vi "Run.vi"(7 "Team Index":i32, 8 "Column":i32, 9 "Row":i32, 10 "View":i32[](array[numeric]) caption="View (Team Index, -1: empty)", 11 "Runner in":refnum<class "Rain.lvclass">) -> (0 "Replicated":refnum<class "Square.lvclass">, 1 "Direction":T1, 2 "Action":T2, 3 "Square Out":refnum<class "Square.lvclass">)   [LabVIEW 2020, in "Rain.lvclass"]
uses:
  Rain.lvclass
  C:/dev/IlluminatedG/sol-squarebattle/Square/Square.lvclass
  Square/Square.lvclass
  Type Defs/Action Enum.ctl
  Type Defs/Direction Enum.ctl
  Common/Attack Options.ctl
  SubVIs/Read-Only Globals.vi
  SubVIs/Globals (private).vi
  Common/Find Enemy.vi
  Common/Reverse Direction.vi
  Common/Common.lvlib
  Type Defs/SB Type Defs.lvlib
panel:
  # "NW\nN\nNE\nE\nSE\nS\nSW\nW"
  # "NOTICE - YOU MUST NOT REMOVE THIS NOTICE. PER THE FOLLOWING LICENSE, YOU MAY REPRODUCE THIS SOFTWARE PROVIDED YOU FOLLOW THE TERMS\nOF THE LICENSE.\n\n---BEGIN BSD LICENSE (http://opensource.org/licenses/BSD-2-Clause)---\nCopyright (c) 2015, Endigit, Inc. <robert@endigit.com>\nAll rights reserved.\n\nRedistribution and use in source and binary forms, with or without modification, are permitted provided that the following conditions are met:\n\n1. Redistributions of source code must retain the above copyright notice, this list of conditions and the following disclaimer.\n\n2. Redistributions in binary form must reproduce the above copyright notice, this list of conditions and the following disclaimer in the documentation and/or other \nmaterials provided with the distribution.\n\nTHIS SOFTWARE IS PROVIDED BY THE COPYRIGHT HOLDERS AND CONTRIBUTORS \"AS IS\" AND ANY EXPRESS OR IMPLIED WARRANTIES, INCLUDING, BUT NOT \nLIMITED TO, THE IMPLIED WARRANTIES OF MERCHANTABILITY AND FITNESS FOR A PARTICULAR PURPOSE ARE DISCLAIMED. IN NO EVENT SHALL THE COPYRIGHT \nHOLDER OR CONTRIBUTORS BE LIABLE FOR ANY DIRECT, INDIRECT, INCIDENTAL, SPECIAL, EXEMPLARY, OR CONSEQUENTIAL DAMAGES (INCLUDING, BUT NOT \nLIMITED TO, PROCUREMENT OF SUBSTITUTE GOODS OR SERVICES; LOSS OF USE, DATA, OR PROFITS; OR BUSINESS INTERRUPTION) HOWEVER CAUSED AND ON \nANY THEORY OF LIABILITY, WHETHER IN CONTRACT, STRICT LIABILITY, OR TORT (INCLUDING NEGLIGENCE OR OTHERWISE) ARISING IN ANY WAY OUT OF THE USE \nOF THIS SOFTWARE, EVEN IF ADVISED OF THE POSSIBILITY OF SUCH DAMAGE.\n---END BSD LICENSE---"
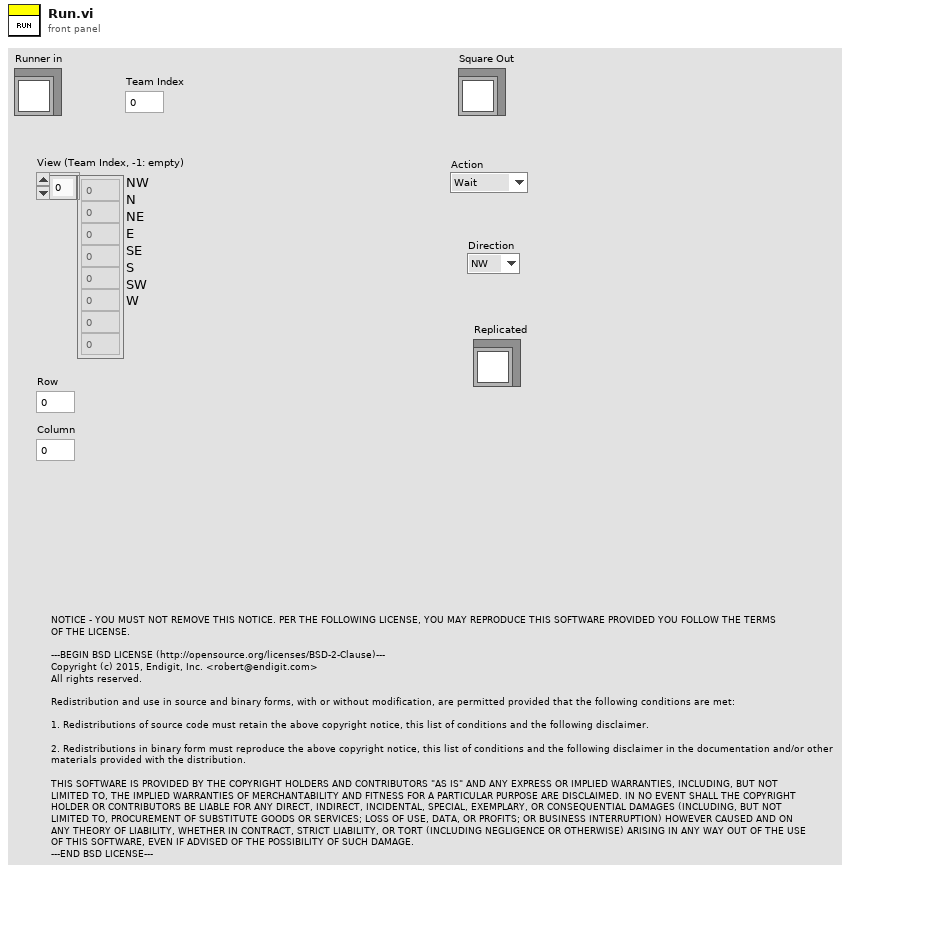
[diagram p1: front panel]
types:
  T1 = typedef "SB Type Defs.lvlib/Direction Enum.ctl" = enum16{"NW", "N", "NE", "E", "SE", "S", "SW", "W"}
  T2 = typedef "SB Type Defs.lvlib/Action Enum.ctl" = enum16{"Wait", "Move", "Attack", "Replicate"}
  T3 = typedef "Common.lvlib/Attack Options.ctl" = enum16{"Attack", "Run", "Distract"}
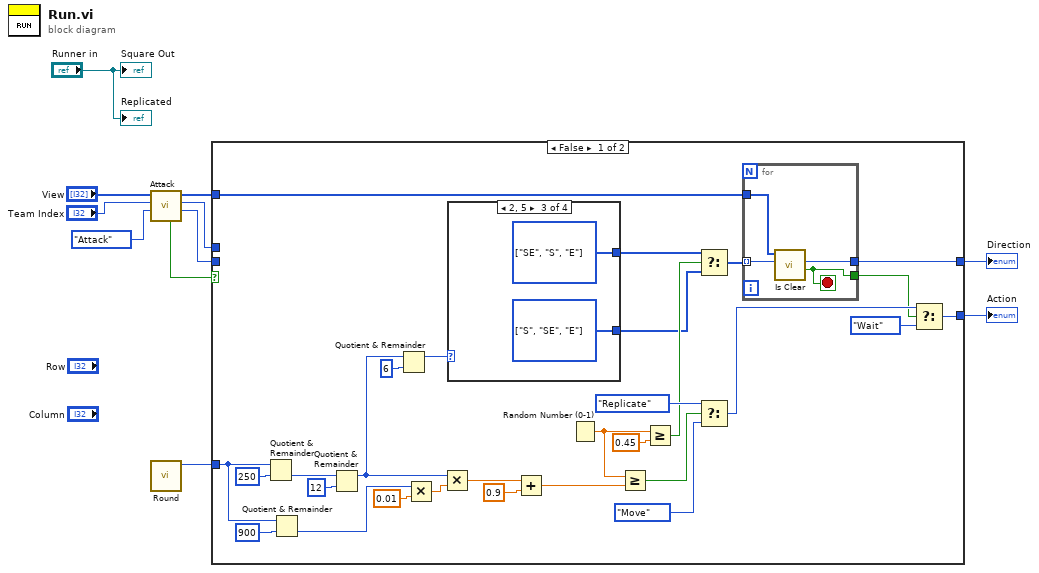
[diagram p0: block diagram]
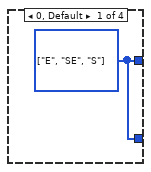
[diagram p2: hidden frame]
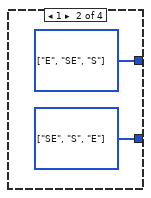
[diagram p3: hidden frame]
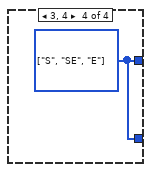
[diagram p4: hidden frame]
diagram:
  n1 = call "Attack.vi"("Attack?"=Attack_Options."Attack" ("Attack"), "Team Index"="Team Index", "View"="View") -> ("Direction"=w10:i32, "Action"=w8:T2, "View"=w6:i32[], "Enemy Found?"=w11:bool)  [unwired: 3 in, 2 out]
  n2 = call "Round.vi"() -> ("Round"=w3:i32)  [unwired: 11 in]
  n3 = case shown="False" w11 {
    tunnel: w10 -> [_ w52]
    tunnel: [w33 w52] -> w9
    tunnel: w8 -> [_ w51]
    tunnel: [w37 w51] -> w7
    tunnel: w6 -> [w34 _]
    tunnel: w3 -> [w16 _]
    frame False {
      n4 = Quotient & Remainder(x=w16, y=250) -> (floor(x/y)=w24:i32)  [unwired: 1 out]
      n5 = Quotient & Remainder(x=w16, y=900) -> (floor(x/y)=w14:i32)  [unwired: 1 out]
      n6 = Quotient & Remainder(x=w24, y=12) -> (x-y*floor(x/y)=w18:i32)  [unwired: 1 out]
      n7 = Quotient & Remainder(x=w18, y=6) -> (x-y*floor(x/y)=w17:i32)  [unwired: 1 out]
      n8 = Multiply(x=w14, y=0.01) -> (x*y=w12:dbl)
      n9 = Multiply(x=w18, y=w12) -> (x*y=w23:dbl)
      n10 = case shown="2, 5" w17 {
        tunnel: [w41 w43 w45 w46] -> w28
        tunnel: [w41 w42 w44 w46] -> w29
        frame 0, Default {
          w41 = T1[] [enum."E", enum."SE", enum."S"] items=["NW", "N", "NE", "E", "SE", "S", "SW", "W"]
        }
        frame 1 {
          w42 = T1[] [enum."SE", enum."S", enum."E"] items=["NW", "N", "NE", "E", "SE", "S", "SW", "W"]
          w43 = T1[] [enum."E", enum."SE", enum."S"] items=["NW", "N", "NE", "E", "SE", "S", "SW", "W"]
        }
        frame 2, 5 {
          w44 = T1[] [enum."S", enum."SE", enum."E"] items=["NW", "N", "NE", "E", "SE", "S", "SW", "W"]
          w45 = T1[] [enum."SE", enum."S", enum."E"] items=["NW", "N", "NE", "E", "SE", "S", "SW", "W"]
        }
        frame 3, 4 {
          w46 = T1[] [enum."S", enum."SE", enum."E"] items=["NW", "N", "NE", "E", "SE", "S", "SW", "W"]
        }
      }
      n11 = Add(x=w23, y=0.9) -> (x+y=w21:dbl)
      n12 = Random Number (0-1)() -> (number: 0 to 1=w26:dbl)
      n13 = Greater Or Equal?(x=w26, y=w21) -> (x >= y?=w32:bool)
      n14 = Greater Or Equal?(x=w26, y=0.45) -> (x >= y?=w30:bool)
      n15 = Select(t=w28, s=w30, f=w29) -> (s? t:f=w27:T1[])
      n16 = Select(t=Action_Enum."Replicate" ("Action"), s=w32, f=Action_Enum."Move" ("Action")) -> (s? t:f=w38:T2)
      n17 = for {
        tunnel: [w48] -> w36
        tunnel: w27 -> [w50] mode=indexing
        tunnel: w34 -> [w49]
        tunnel: [w47] -> w33
        stop <- w48 stop-if-true
        n18 = call "Is Clear.vi"("Direction"=w50, "Maze"=w49) -> ("Can Move?"=w48:bool, "Direction Out"=w47:T1)  [unwired: 7 in, 1 out]
      }
      n19 = Select(t=w38, s=w36, f=Action_Enum."Wait" ("Action")) -> (s? t:f=w37:T2)
    }
    frame True {
    }
  }
  "Action" <- w7
  "Direction" <- w9
  "Square Out" <- "Runner in"
  "Replicated" <- "Runner in"
